vi "4145 Data Output.vi"(0 "4145_GPIB_Param":T1={"Address_string"="17", "timeout ms"=25000, "Terminator"=",", "LoggerQueue"=refnum}, 5 "name":string, 11 "error in":T2) -> (4 "4145_GPIB_COM_OUT":T1={"Address_string"="17", "timeout ms"=25000, "Terminator"=",", "LoggerQueue"=refnum}, 6 "headings OUT":string[](array[string]), 8 "read data array OUT":dbl[](array[numeric]) format="%^.2e", 15 "error out":T2)   [LabVIEW 2014]
doc: "This VI sends the data output command to the instrument, directing the instrument to send all the data from the specified channel to the controller via GPIB. Be sure the delimiter (bit switch 6 on the GP-IB Control Switch (Figure 3-50), is set at the factory to comma (,)), is a comma."
uses:
  typedef/4145_GPIB_Com.ctl
  typedef/4145_que_msg.ctl
  typedef/4145 command enum.ctl
panel:
  out "string output":string
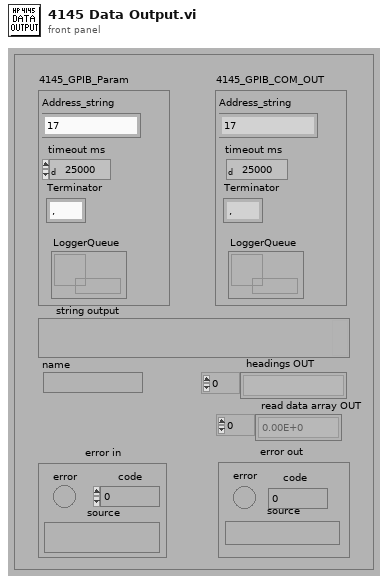
[diagram p1: front panel]
types:
  T1 = typedef "4145_GPIB_Com.ctl" = cluster{"Address_string":string, "timeout ms":u32, "Terminator":string, "LoggerQueue":refnum<queue>}
  T2 = cluster{"error":bool, "code":i32, "source":string}
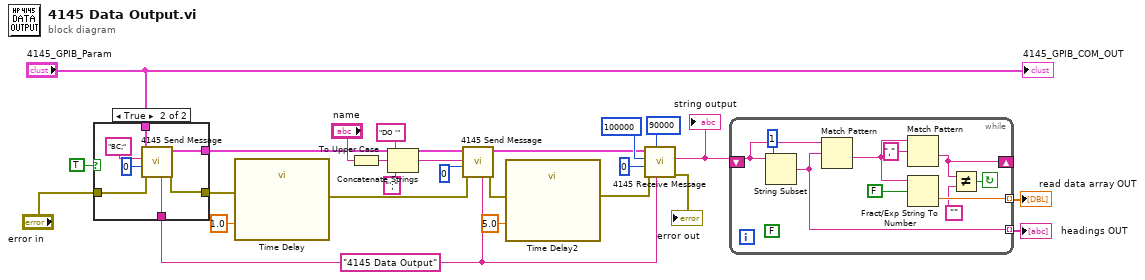
[diagram p0: block diagram]
diagram:
  w2 = "4145 Data Output"
  n1 = case shown="True" TRUE {
    tunnel: "error in" -> [w27 w33]
    tunnel: [w27 w30] -> w14
    tunnel: "4145_GPIB_Param" -> [w26 w32]
    tunnel: w2 -> [_ w29]
    tunnel: [w26 w28] -> w3
    frame False {
    }
    frame True {
      n2 = call "4145 Send Message.vi"("source IN"=w29, "error in"=w33, "write mode (set END:0)"=0, "write buffer IN"="BC;", "4145_GPIB_COM_IN"=w32) -> ("error out"=w30:T2, "4145_GPIB_COM_OUT"=w28:T1)  [unwired: 3 in, 2 out]
    }
  }
  n3 = call "Time Delay"("error in (no error)"=w14, "Delay Time (s)"=1.0) -> ("error out"=w13:errorcluster)  [unwired: 9 in]
  n4 = To Upper Case(1:"name") -> (0:w1:string)
  n5 = Concatenate Strings("DO '", w1, "';") -> (w23:string)
  n6 = call "4145 Send Message.vi"("source IN"=w2, "error in"=w13, "write mode (set END:0)"=0, "write buffer IN"=w23, "4145_GPIB_COM_IN"=w3) -> ("error out"=w9:T2, "4145_GPIB_COM_OUT"=w5:T1)  [unwired: 3 in, 2 out]
  n7 = call "Time Delay2"("error in (no error)"=w9, "Delay Time (s)"=5.0) -> ("error out"=w12:errorcluster)  [unwired: 9 in]
  n8 = call "4145 Receive Message.vi"("source"=w2, "timeout ms"=90000, "error in"=w12, "read mode"=0, "byte count in"=100000, "4145_GPIB_COM_ctrl"=w5) -> ("error out"=→"error out":T2, "read buffer OUT"=w6:string)  [unwired: 1 in, 2 out]
  "string output" <- w6
  n9 = while {
    tunnel: [w36] -> w19 mode=indexing
    tunnel: [w44] -> w20 mode=indexing
    shift-left: w6 -> [w43]
    shift-right: [w39] -> _
    stop <- w37 continue-if-true
    (unwired) FALSE ("use system decimal point (T)")
    n10 = String Subset(string=w43, length (rest)=1) -> (substring=w36:string)  [unwired: 1 in]
    n11 = Match Pattern(string=w43, regular expression=w36) -> (after substring=w41:string)  [unwired: 1 in, 3 out]
    n12 = Match Pattern(string=w41, regular expression=",") -> (after substring=w39:string)  [unwired: 1 in, 3 out]
    n13 = Fract/Exp String To Number(use system decimal point (T)=FALSE, string=w41) -> (number=w44:dbl)  [unwired: 2 in, 1 out]
    n14 = Not Equal?(x=w39, y="") -> (x != y?=w37:bool)
  }
  "read data array OUT" <- w20
  "headings OUT" <- w19
  "4145_GPIB_COM_OUT" <- "4145_GPIB_Param"
